vi "Write.vi"(8 "error in (no error)":errorcluster, 9 "Variant":variant, 10 "String":string, 11 "RS232 to GPIB ConvBox in":refnum<class "RS-xxx to GPIB ConvBox.lvclass">) -> (0 "error out":errorcluster, 3 "RS232 to GPIB ConvBox out":refnum<class "RS-xxx to GPIB ConvBox.lvclass">)   [LabVIEW 2018, in "Protocols.lvlib" / "RS-xxx to GPIB ConvBox.lvclass"]
uses:
  RS-xxx to GPIB ConvBox.lvclass
  RS-xxx to GPIB ConvBox.lvclass/RS-xxx to GPIB ConvBox.ctl
  Data Access/Read Port Ref.vi
  Data Access/Read GPIB Address.vi
  Data Access/Write Port Ref.vi
  <vilib>/dlg_ctls.llb/Space Constant.vi
  SubVIs/Status ConvBox.vi
  SubVIs/CheckListener ConvBox.vi
  <vilib>/Utility/error.llb/Clear Errors.vi
  <vilib>/Utility/error.llb/Error Cluster From Error Code.vi
  Protocol Parent/Protocol Parent.lvclass
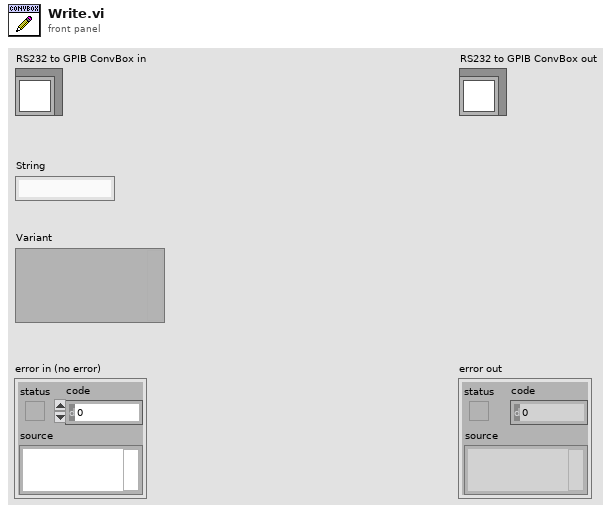
[diagram p1: front panel]
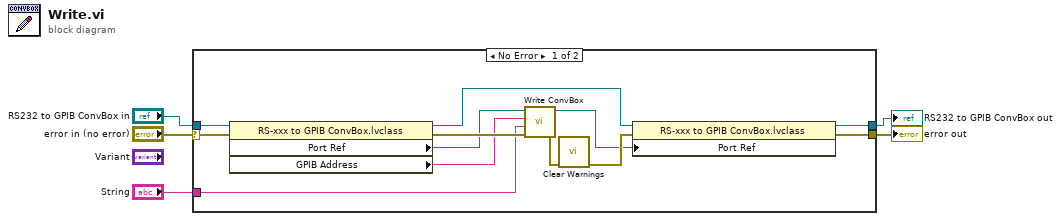
[diagram p0: block diagram]
diagram:
  n1 = case shown="No Error" "error in (no error)" {
    selector: "error in (no error)" -> [w11 w19]
    tunnel: "RS232 to GPIB ConvBox in" -> [w17 w18]
    tunnel: "String" -> [w7 _]
    tunnel: [w14 w19] -> w4
    tunnel: [w12 w18] -> w3
    frame No Error {
      n2 = property class="RS-xxx to GPIB ConvBox.lvclass"(reference=w17, error in=w11) -> (reference out=w13:refnum<class "RS-xxx to GPIB ConvBox.lvclass">, error out=w16:errorcluster, "Port Ref"=w15:refnum<visa-resource-name>, "GPIB Address"=w6:string)
      n3 = call "Write ConvBox.vi"("error in"=w16, "data"=w7, "address string"=w6, "VISA resource in"=w15) -> ("error out"=w10:errorcluster, "VISA resource out"=w8:refnum<visa-resource-name>)  [unwired: 5 in, 1 out]
      n4 = call "Clear Warnings.vi"("error in (no error)"=w10) -> ("error out"=w9:errorcluster)  [unwired: 10 in]
      n5 = property class="RS-xxx to GPIB ConvBox.lvclass"(reference=w13, error in=w9, "Port Ref"=w8) -> (reference out=w12:refnum<class "RS-xxx to GPIB ConvBox.lvclass">, error out=w14:errorcluster)
    }
    frame Error {
    }
  }
  "error out" <- w4
  "RS232 to GPIB ConvBox out" <- w3
